vi "CMI ADS127L21 - Try Fetch Data.vi"(8 "error in (no error)":errorcluster, 11 "ADS127L21 session":T2 {"channels"."Channel" min=1 max=8 step=1}) -> (0 "error out":errorcluster, 2 "data":T1, 3 "ADS127L21 session out":T2 {"channels"."Channel" min=1 max=8 step=1})   [LabVIEW 2020]
uses:
  CMI ADS127L21 - Session.ctl
  CMI ADS127L21 - Record Channel.ctl
  CMI ADS127L21 - Input Range.ctl
  CMI ADS127L21 - Input Mode.ctl
  CMI ADS127L21 - Input Impedance.ctl
  CMI ADS127L21 - EXTOUT Mode.ctl
  CMI ADS127L21 - EXTOUT Polarity.ctl
  CMI ADS127L21 - Fetch Data.ctl
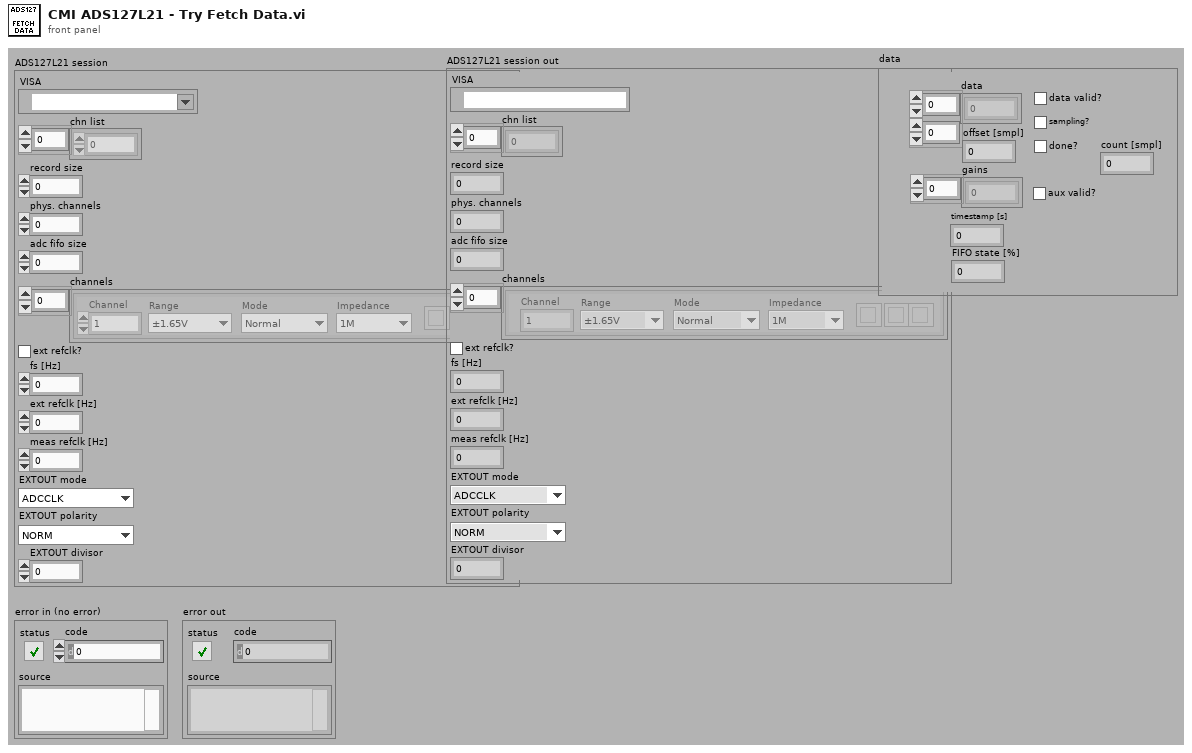
[diagram p1: front panel]
types:
  T1 = typedef "CMI ADS127L21 - Fetch Data.ctl" = cluster{"data":i32[][], "data valid?":bool, "sampling?":bool, "done?":bool, "gains":dbl[], "aux valid?":bool, "timestamp [s]":dbl, "FIFO state [%]":dbl, "offset [smpl]":i32, "count [smpl]":i32}
  T2 = typedef "CMI ADS127L21 - Session.ctl" = cluster{"VISA":refnum<visa-resource-name>, "chn list":i32[], "record size":i32, "phys. channels":i32, "adc fifo size":i32, "channels":T3[], "ext refclk?":bool, "fs [Hz]":dbl, "ext refclk [Hz]":dbl, "meas refclk [Hz]":dbl, "EXTOUT mode":T7, "EXTOUT polarity":T8, "EXTOUT divisor":i32}
  T3 = typedef "CMI ADS127L21 - Record Channel.ctl" = cluster{"Range":T4, "Channel":i32, "Mode":T5, "Impedance":T6, "btn clr":bool, "btn up":bool, "btn down":bool}
  T4 = typedef "CMI ADS127L21 - Input Range.ctl" = enum16{"±1.65V", "±2V"}
  T5 = typedef "CMI ADS127L21 - Input Mode.ctl" = enum16{"Normal", "Inverted", "GND"}
  T6 = typedef "CMI ADS127L21 - Input Impedance.ctl" = enum16{"1M", "1k5"}
  T7 = typedef "CMI ADS127L21 - EXTOUT Mode.ctl" = enum16{"ADCCLK", "REFCLK", "SMPLCLK", "FIRST"}
  T8 = typedef "CMI ADS127L21 - EXTOUT Polarity.ctl" = enum16{"NORM", "INV"}
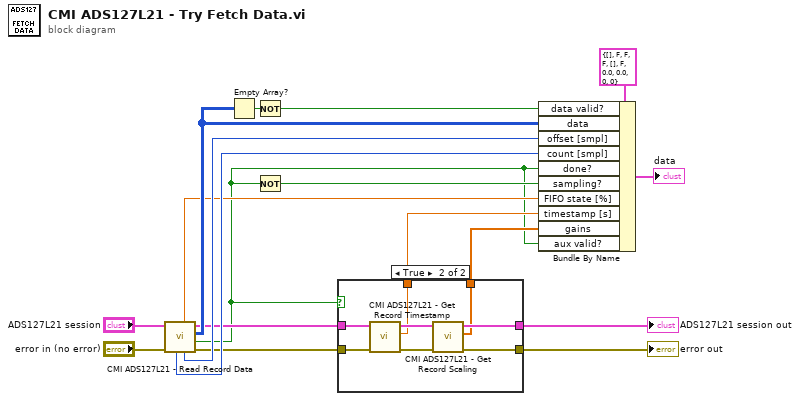
[diagram p0: block diagram]
diagram:
  n1 = call "CMI ADS127L21 - Read Record Data.vi"("error in (no error)"="error in (no error)", "session in"="ADS127L21 session") -> ("error out"=w8:errorcluster, "done?"=w2:bool, "Raw Sample Data (column per channel)"=w12:i32[][], "session out"=w7:T2, "sample offset"=w15:i32, "FIFO usage [%]"=w9:dbl, "sample count"=w11:i32)  [unwired: 3 in]
  n2 = Empty Array?(array=w12) -> (empty?=w14:bool)
  n3 = Not(x=w14) -> (.not. x?=w13:bool)
  n4 = Not(x=w2) -> (.not. x?=w10:bool)
  n5 = case shown="True" w2 {
    tunnel: w8 -> [w19 w28]
    tunnel: w7 -> [w20 w26]
    tunnel: [w20 w24] -> w6
    tunnel: [w19 w23] -> w5
    tunnel: [_ w22] -> w4
    tunnel: [_ w21] -> w3
    frame False {
    }
    frame True {
      n6 = call "CMI ADS127L21 - Get Record Timestamp.vi"("error in (no error)"=w28, "session in"=w26) -> ("error out"=w27:errorcluster, "timestamp [s]"=w22:ext, "session out"=w25:T2)  [unwired: 7 in]
      n7 = call "CMI ADS127L21 - Get Record Scaling.vi"("error in (no error)"=w27, "session in"=w25) -> ("error out"=w23:errorcluster, "Gain (one value per channel)"=w21:dbl[], "session out"=w24:T2)  [unwired: 7 in]
    }
  }
  "error out" <- w5
  "ADS127L21 session out" <- w6
  n8 = Bundle By Name(cluster=T1 {"data"=[], "data valid?"=FALSE, "sampling?"=FALSE, "done?"=FALSE, "gains"=[], "aux valid?"=FALSE, "timestamp [s]"=0.0, "FIFO state [%]"=0.0, "offset [smpl]"=0, "count [smpl]"=0} ("data"), "data valid?"=w13, "data"=w12, "offset [smpl]"=w15, "count [smpl]"=w11, "done?"=w2, "sampling?"=w10, "FIFO state [%]"=w9, "timestamp [s]"=w4, "gains"=w3, "aux valid?"=w2) -> (→"data":T1)
